vi "RSZVB Trace Evaluation Range.vi"(6 "Start (300.0e3 Hz)":dbl=300000.0 format="%^.3e", 7 "Stop (4.0e9 Hz)":dbl=4000000000.0 format="%^.3e", 8 "error in (no error)":errorcluster {"code" format="%.0x"}, 9 "Evaluation Range (0: Full Span)":i32(ring) items=["Full Span", "Range 1", "Range 2", "Range 3", "Range 4", "Range 5", "Range 6", "Range 7", "Range 8", "Range 9", "Range 10"], 10 "Channel (Trace) (1)":i32=1, 11 "VISA session":refnum<visa-resource-name>) -> (0 "error out":errorcluster {"code" format="%.0x"}, 3 "dup VISA session":refnum<visa-resource-name>)   [LabVIEW 2011]
doc: "This VI define the range for the statistical and phase evaluation. The evaluation range is a continuous interval of the sweep variable.\n\nIt is possible to define and select up to ten different evaluation ranges for each setup. Full Span means that the search range is equal to the sweep range. The statistical and phase evaluation takes into account all measurement points with stimulus values xi between the Start and Stop value of the evaluation range:\n\n Start <= xi <= Stop\n\nRemote-control command(s):\nCALCulate<Ch/Tr>:STATistics:DOMain:USER <numeric_value>\nCALCulate<Ch/Tr>:STATistics:DOMain:USER:STARt <numeric_value>\nCALCulate<Ch/Tr>:STATistics:DOMain:USER:STOP <numeric_value>"
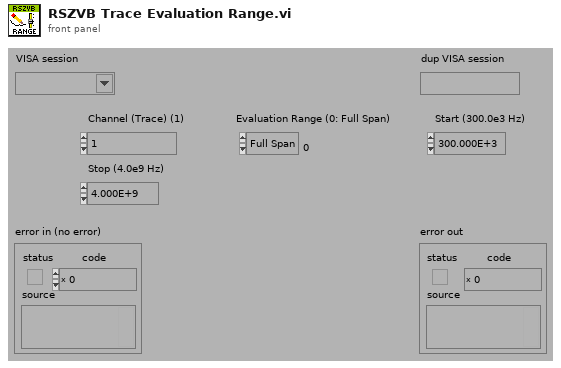
[diagram p1: front panel]
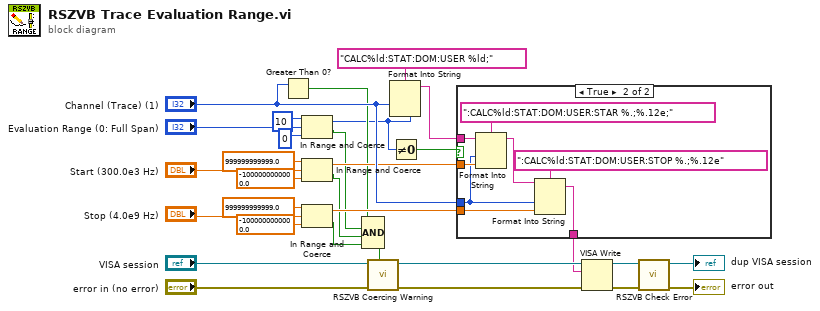
[diagram p0: block diagram]
diagram:
  n1 = Greater Than 0?(x="Channel (Trace) (1)") -> (x > 0?=w8:bool)
  n2 = In Range and Coerce(upper limit=10, x="Evaluation Range (0: Full Span)", lower limit=0) -> (coerced(x)=w1:i32, In Range?=w7:bool)
  n3 = In Range and Coerce(upper limit=999999999999.0, x="Start (300.0e3 Hz)", lower limit=-1000000000000.0) -> (coerced(x)=w10:dbl, In Range?=w6:bool)
  n4 = In Range and Coerce(upper limit=999999999999.0, x="Stop (4.0e9 Hz)", lower limit=-1000000000000.0) -> (coerced(x)=w9:dbl, In Range?=w5:bool)
  n5 = Compound Arithmetic op=AND(w8, w7, w6, w5) -> (w4:bool)
  n6 = call "RSZVB Coercing Warning.vi"("In Range?"=w4, "error in (no error)"="error in (no error)", "VISA session"="VISA session") -> ("error out"=w29:errorcluster, "dup VISA session"=w30:refnum<visa-resource-name>)  [unwired: 7 in]
  n7 = Format Into String(format string="CALC%ld:STAT:DOM:USER %ld;", "Channel (Trace) (1)", w1) -> (resulting string=w12:string)  [unwired: 2 in, 1 out]
  n8 = Not Equal To 0?(x=w1) -> (x != 0?=w2:bool)
  n9 = case shown="True" w2 {
    tunnel: [w31 w38] -> w26
    tunnel: w12 -> [w31 w36]
    tunnel: "Channel (Trace) (1)" -> [_ w32]
    tunnel: w10 -> [_ w34]
    tunnel: w9 -> [_ w33]
    frame False {
    }
    frame True {
      n10 = Format Into String(format string=":CALC%ld:STAT:DOM:USER:STAR %.;%.12e;", initial string=w36, w32, w34) -> (resulting string=w35:string)  [unwired: 1 in, 1 out]
      n11 = Format Into String(format string=":CALC%ld:STAT:DOM:USER:STOP %.;%.12e", initial string=w35, w32, w33) -> (resulting string=w38:string)  [unwired: 1 in, 1 out]
    }
  }
  n12 = VISA Write(VISA resource name=w30, write buffer=w26, error in (no error)=w29) -> (VISA resource name out=w27:refnum<visa-resource-name>, error out=w28:errorcluster)  [unwired: 1 out]
  n13 = call "RSZVB Check Error.vi"("error in (no error)"=w28, "VISA session"=w27) -> ("error out"=→"error out":errorcluster, "dup VISA session"=→"dup VISA session":refnum<visa-resource-name>)  [unwired: 8 in]
